vi "test_Generator - Host to FPGA.vi"(8 "error in (no error)":errorcluster, 10 "IO Lines Patttern":T1[](array[typedef]) {"Duration (us)" min=0.005 max=42550000.0 step=0.005 format="%#.3f"}, 11 "IO Lines Enable":T2={"Enable"=[FALSE, FALSE, FALSE, FALSE, FALSE, FALSE, FALSE, FALSE, FALSE, FALSE, FALSE, FALSE, FALSE, FALSE, FALSE, FALSE, FALSE, FALSE, FALSE, FALSE, FALSE, FALSE, FALSE, FALSE, FALSE, FALSE, FALSE, FALSE, FALSE, FALSE, FALSE, FALSE]}) -> (0 "error out":errorcluster, 2 "IO Data_Wr":u32[](array[numeric]) format="%.0x", 3 "IO Data_Dir":u32 format="%.0x")   [LabVIEW 2016]
uses:
  Host/Typedefs/IO Lines Enable.ctl
  Host/Typedefs/IO Lines State.ctl
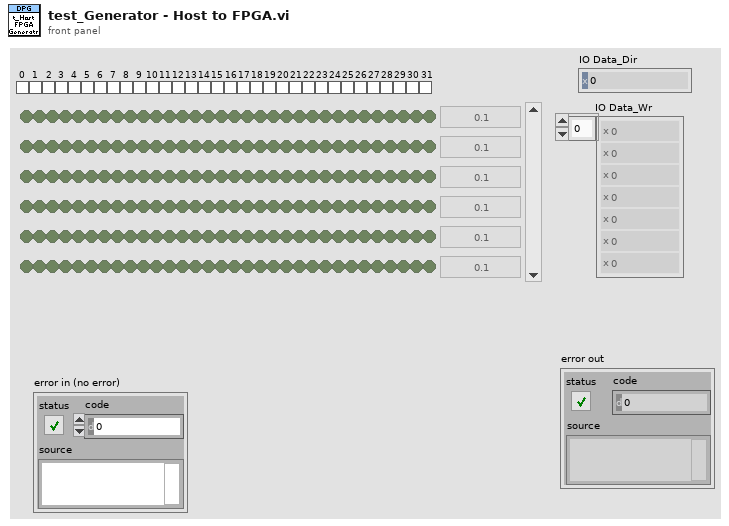
[diagram p1: front panel]
types:
  T1 = typedef "IO Lines State.ctl" = cluster{"State":bool[], "Duration (us)":dbl}
  T2 = typedef "IO Lines Enable.ctl" = cluster{"Enable":bool[]}
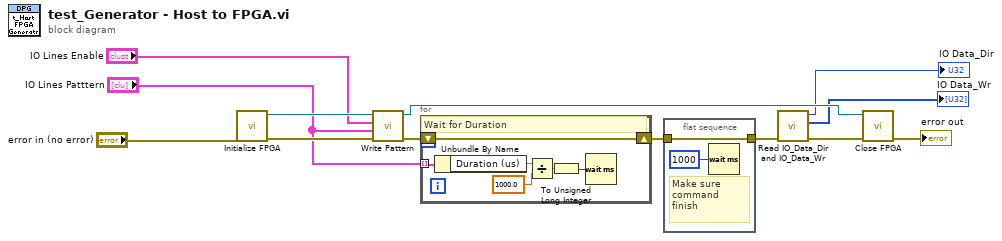
[diagram p0: block diagram]
diagram:
  n1 = call "Initialize FPGA.vi"("error in (no error)"="error in (no error)") -> ("error out"=w13:errorcluster, "FPGA VI Reference"=w12:refnum<k20>)  [unwired: 9 in]
  n2 = call "Write Pattern.vi"("error in (no error)"=w13, "IO Lines Pattteen"="IO Lines Patttern", "IO Lines Enable"="IO Lines Enable", "Refnum in"=w12) -> ("error out"=w8:errorcluster, "FPGA VI Reference Out"=w10:refnum<k20>)  [unwired: 5 in, 1 out]
  n3 = for {
    tunnel: "IO Lines Patttern" -> [w19] mode=indexing
    shift-right: [w14] -> w5
    shift-left: w8 -> [w14]
    # "Wait for Duration"
    n4 = Unbundle By Name(w19) -> ("Duration (us)"=w18:dbl)
    n5 = Divide(x=w18, y=1000.0) -> (x/y=w16:dbl)
    n6 = To Unsigned Long Integer(number=w16) -> (unsigned 32bit integer=w15:u32)
    n7 = Wait (ms)(milliseconds to wait=w15) -> ()  [unwired: 1 out]
  }
  n8 = flat-sequence {
    tunnel: w5 -> [w20]
    tunnel: [w20] -> w3
    frame #0 {
      # "Make sure \ncommand \nfinish"
      n9 = Wait (ms)(milliseconds to wait=u32 1000) -> ()  [unwired: 1 out]
    }
  }
  n10 = call "Read IO_Data_Dir and IO_Data_Wr.vi"("error in (no error)"=w3) -> ("error out"=w2:errorcluster, "IO Data_Wr"=→"IO Data_Wr":u32[], "IO Data_Dir"=→"IO Data_Dir":u32)  [unwired: 8 in]
  n11 = call "Close FPGA.vi"("error in (no error)"=w2, "Refnum in"=w10) -> ("error out"=→"error out":errorcluster)  [unwired: 9 in]
